vi "CRYLogin Write Config.vi"(6 "User Name In":string, 8 "Remember In":bool, 9 "Password  In":T1, 10 "Level In":enum16{"engr", "tech", "oper"}(ring), 11 "Login Section In":cluster{"Key":string, "Value":string}[](array[cluster])) -> ()   [LabVIEW 2013]
panel:
  # "CRYSoundLab Login Write Configure"
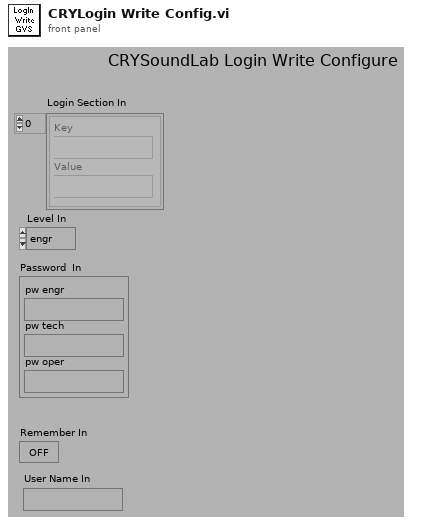
[diagram p1: front panel]
types:
  T1 = cluster{"pw engr":string, "pw tech":string, "pw oper":string}
  T2 = cluster{"Section":string, "Item":cluster{"Key":string, "Value":string}[]}
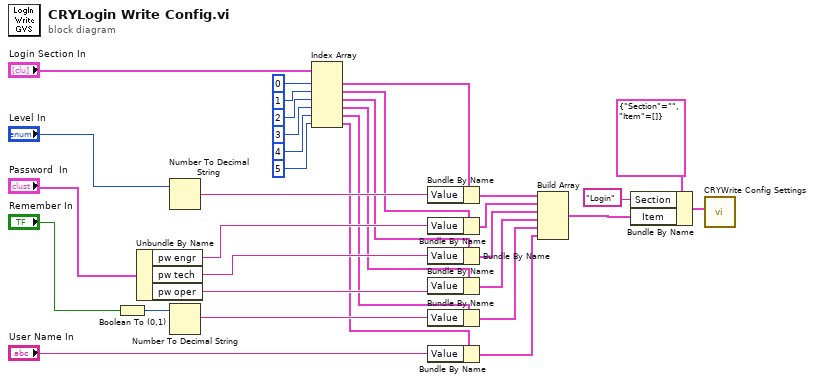
[diagram p0: block diagram]
diagram:
  n1 = Boolean To (0,1)(Boolean="Remember In") -> (0, 1=w33:i16)
  n2 = Unbundle By Name("Password  In") -> ("pw engr"=w24:string, "pw tech"=w21:string, "pw oper"=w18:string)
  n3 = Number To Decimal String(number="Level In") -> (decimal integer string=w27:string)  [unwired: 1 out]
  n4 = Number To Decimal String(number=w33) -> (decimal integer string=w16:string)  [unwired: 1 out]
  n5 = Index Array(array="Login Section In", index #1=0 ("index"), index #2=1 ("index"), index #3=2 ("index"), index #4=3 ("index"), index #5=4 ("index"), index #6=5 ("index")) -> (element #1=w28:cluster{"Key":string, "Value":string}, element #2=w26:cluster{"Key":string, "Value":string}, element #3=w22:cluster{"Key":string, "Value":string}, element #4=w19:cluster{"Key":string, "Value":string}, element #5=w17:cluster{"Key":string, "Value":string}, element #6=w13:cluster{"Key":string, "Value":string})
  n6 = Bundle By Name(cluster=w28, "Value"=w27) -> (w11:cluster{"Key":string, "Value":string})
  n7 = Bundle By Name(cluster=w26, "Value"=w24) -> (w10:cluster{"Key":string, "Value":string})
  n8 = Bundle By Name(cluster=w22, "Value"=w21) -> (w9:cluster{"Key":string, "Value":string})
  n9 = Bundle By Name(cluster=w19, "Value"=w18) -> (w8:cluster{"Key":string, "Value":string})
  n10 = Bundle By Name(cluster=w17, "Value"=w16) -> (w7:cluster{"Key":string, "Value":string})
  n11 = Bundle By Name(cluster=w13, "Value"="User Name In") -> (w6:cluster{"Key":string, "Value":string})
  n12 = Build Array(w11, w10, w9, w8, w7, w6) -> (w5:cluster{"Key":string, "Value":string}[])
  n13 = Bundle By Name(cluster=T2 {"Section"="", "Item"=[]}, "Section"="Login", "Item"=w5) -> (w2:T2)
  n14 = call "CRYWrite Config Settings.vi"("Config Data"=w2) -> ()  [unwired: 1 in, 8 out]
